vi "RB2 find blue 2 dot.vi"(0 "Image In":T1, 1 "error in":errorcluster) -> (2 "Image Out":T1, 3 "Num of\nBlue Dots":i32, 4 "Blue Dot\nLocation":T2(array[cluster]), 5 "error out":errorcluster)   [LabVIEW 2012]
doc: "This VI find a Blue dot on the vehicle in the Mars landscape for Robotics II Spring 2014. It reports the number of Blue dots found and their location."
uses:
  <vilib>/vision/Image Controls.llb/IMAQ Image.ctl
  <vilib>/vision/NI_Vision_Development_Module.lvlib
panel:
  out "Mars Result":T1(plugin-control)
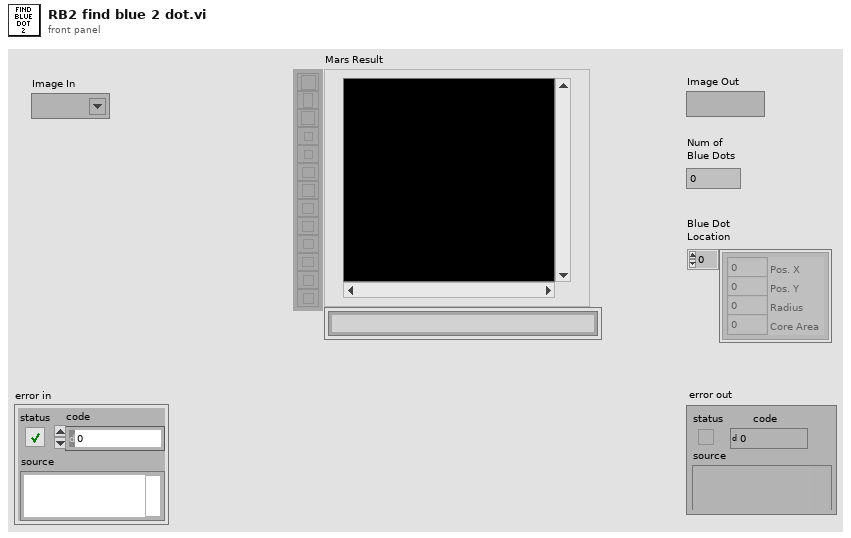
[diagram p1: front panel]
types:
  T1 = typedef "IMAQ Image.ctl" = refnum<image>
  T2 = cluster{"Pos. X":i32, "Pos. Y":i32, "Radius":i32, "Core Area":i32}[]
  T3 = enum32{"AutoM", "Close", "Dilate", "Erode", "Gradient", "Gradient in", "Gradient out", "HitMiss", "Open", "PClose", "POpen", "Thick", "Thin"}
  T4 = typedef "Image Type" = u32
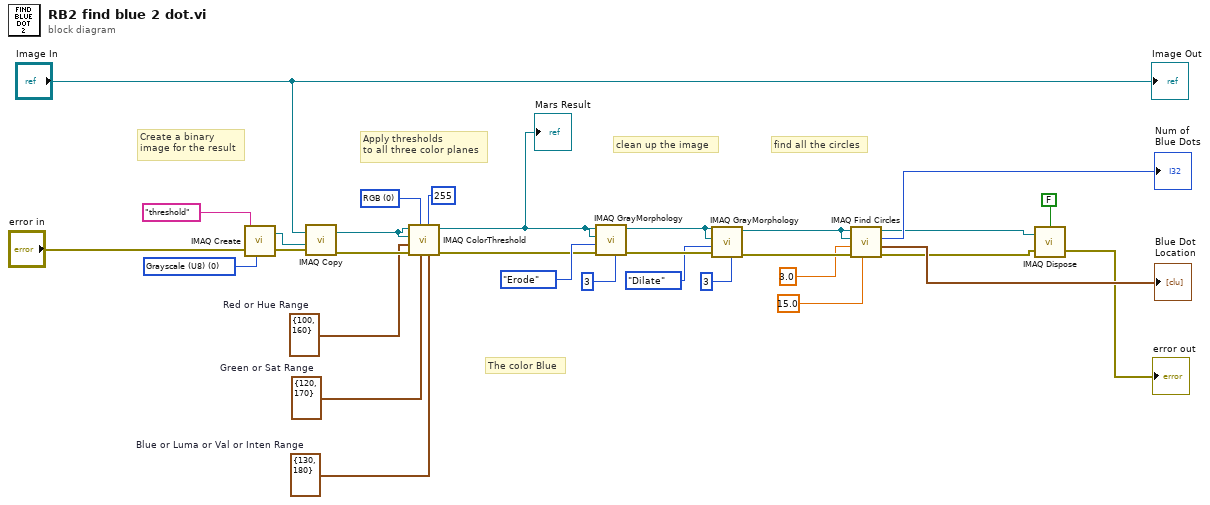
[diagram p0: block diagram]
diagram:
  w1 = cluster{"Lower value":i32, "Upper value":i32} {"Lower value"=130, "Upper value"=180}  # Blue or Luma or Val or Inten Range
  w2 = cluster{"Lower value":i32, "Upper value":i32} {"Lower value"=120, "Upper value"=170}  # Green or Sat Range
  w3 = cluster{"Lower value":i32, "Upper value":i32} {"Lower value"=100, "Upper value"=160}  # Red or Hue Range
  w14 = u16 0 items=["RGB", "HSL", "HSV", "HSI"] ("Color Mode")
  w28 = T4 0 items=["Grayscale (U8)", "Grayscale (I16)", "Grayscale (SGL)", "Complex (CSG)", "RGB (U32)", "HSL (U32)", "RGB (U64)", "Grayscale (U16)"] ("Image Type")
  # "Create a binary\nimage for the result"
  # "The color Blue"
  # "Apply thresholds\nto all three color planes"
  # "find all the circles"
  # "clean up the image"
  n1 = call "IMAQ Create"("Image Name"="threshold", "Image Type"=w28, "error in (no error)"="error in") -> ("New Image"=w30:T1, "error out"=w29:errorcluster)  [unwired: 2 in]
  n2 = call "IMAQ Copy"("error in (no error)"=w29, "Image Dst"=w30, "Image Src"="Image In") -> ("error out"=w15:errorcluster, "Image Dst Out"=w11:T1)  [unwired: 3 in]
  n3 = call "IMAQ ColorThreshold"("Blue or Luma or Val or Inten Range"=w1, "Replace Value"=255, "Green or Sat Range"=w2, "Color Mode"=w14, "error in (no error)"=w15, "Red or Hue Range"=w3, "Image Dst"=w11, "Image Src"=w11) -> ("error out"=w10:errorcluster, "Image Dst Out"=w12:T1)  [unwired: 2 in]
  "Mars Result" <- w12
  n4 = call "IMAQ GrayMorphology"("Number of iterations (1)"=3, "error in (no error)"=w10, "Operation"=T3."Erode", "Image Dst"=w12, "Image Src"=w12) -> ("error out"=w25:errorcluster, "Image Dst Out"=w23:T1)  [unwired: 5 in]
  n5 = call "IMAQ GrayMorphology"("Number of iterations (1)"=3, "error in (no error)"=w25, "Operation"=T3."Dilate", "Image Dst"=w23, "Image Src"=w23) -> ("error out"=w20:errorcluster, "Image Dst Out"=w21:T1)  [unwired: 5 in]
  n6 = call "IMAQ Find Circles"("Max Radius"=sgl 15.0, "error in (no error)"=w20, "Min Radius"=sgl 3.0, "Image Dst"=w21, "Image Src"=w21) -> ("error out"=w7:errorcluster, "Circles Data"=→"Blue Dot\nLocation":T2, "Nb Circles"=→"Num of\nBlue Dots":i32, "Image Dst Out"=w6:T1)  [unwired: 3 in]
  n7 = call "IMAQ Dispose"("All Images? (No)"=FALSE, "Image"=w6, "error in (no error)"=w7) -> ("error out"=→"error out":errorcluster)  [unwired: 3 in]
  "Image Out" <- "Image In"
